vi "Transform.vi"(8 "error in (no error)":errorcluster caption="entrée d'erreur (pas d'erreur)", 9 "y":string[][](array[string]), 10 "X":string[][](array[string]), 11 "PowerTransformer.lvclass":refnum<class "PowerTransformer.lvclass">) -> (0 "error out":errorcluster caption="sortie d'erreur", 2 "Data":T1, 3 "PowerTransformer.lvclass":refnum<class "PowerTransformer.lvclass">)   [LabVIEW 2020, in "PowerTransformer.lvclass"]
doc: "Apply the power transform to each feature using the fitted lambdas.\n\nReturns : \n\n- X_trans : array-like, shape (n_samples, n_features)\nThe transformed data."
uses:
  PowerTransformer.lvclass
  PowerTransformer.lvclass/PowerTransformer.ctl
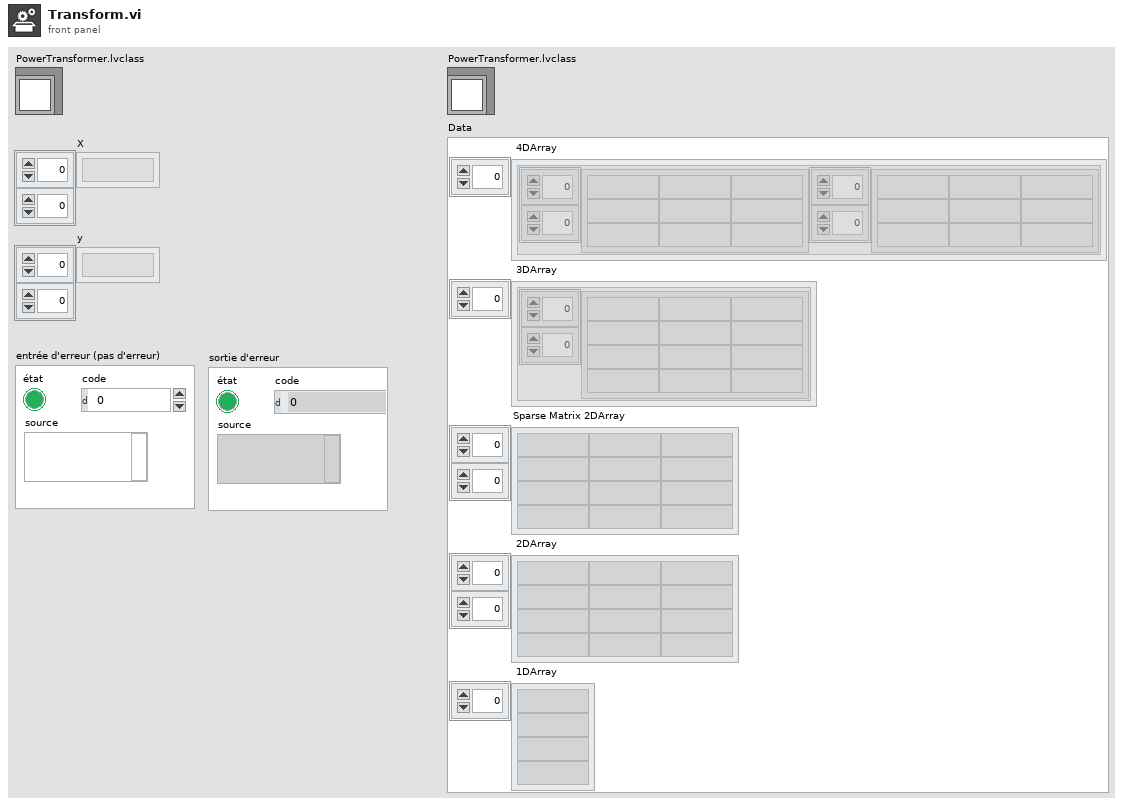
[diagram p1: front panel]
types:
  T1 = cluster{" 4DArray":cluster{"1":string[][], "2":string[][]}[], " 3DArray":cluster{"Tableau":string[][]}[], "Sparse Matrix 2DArray":string[][], " 2DArray":string[][], " 1DArray":string[]}
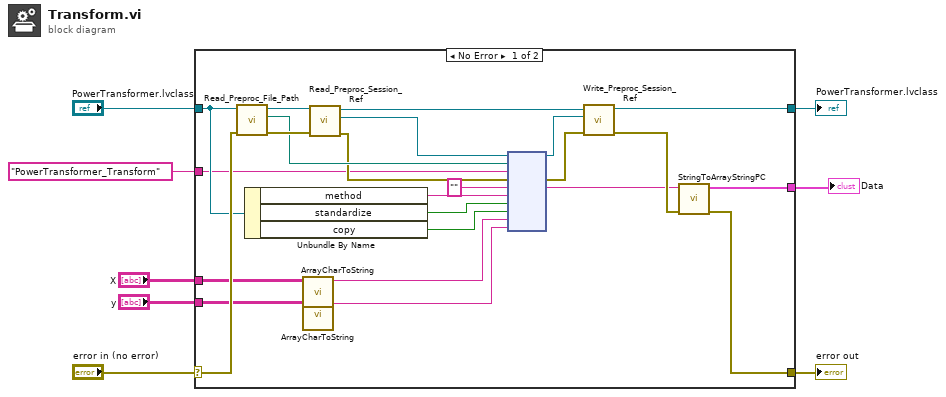
[diagram p0: block diagram]
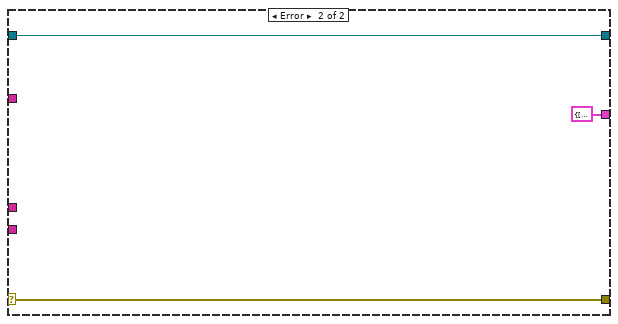
[diagram p2: hidden frame]
diagram:
  n1 = case shown="No Error" "error in (no error)" {
    selector: "error in (no error)" -> [w20 w35]
    tunnel: [w9 w35] -> w7
    tunnel: [w13 w34] -> w5
    tunnel: "PowerTransformer.lvclass" -> [w19 w34]
    tunnel: "PowerTransformer_Transform" ("Fonction") -> [w18 _]
    tunnel: [w10 T1 {" 4DArray"=[], " 3DArray"=[], "Sparse Matrix 2DArray"=[], " 2DArray"=[], " 1DArray"=[]} ("Data")] -> w3
    tunnel: "X" -> [w17 _]
    tunnel: "y" -> [w16 _]
    frame No Error {
      n2 = call-dynamic "Read_Preproc_File_Path.vi"("error in (no error)"=w20, "Python in"=w19) -> ("error out"=w31:errorcluster, "File_Path"=w28:path, "Python out"=w32:refnum<class "PowerTransformer.lvclass">)  [unwired: 7 in]
      n3 = Unbundle By Name(w19) -> ("method"=w23:string, "standardize"=w22:bool, "copy"=w21:bool)
      n4 = call "ArrayCharToString.vi"("TAB"=w17) -> ("Instruction"=w15:string)  [unwired: 10 in]
      n5 = call "ArrayCharToString.vi"("TAB"=w16) -> ("Instruction"=w14:string)  [unwired: 10 in]
      n6 = call-dynamic "Read_Preproc_Session_Ref.vi"("error in (no error)"=w31, "Python in"=w32) -> ("error out"=w27:errorcluster, "Session_ref"=w29:refnum<k35>, "Python out"=w30:refnum<class "PowerTransformer.lvclass">)  [unwired: 7 in]
      n7 = node(w29, w28, w18, w27, "", w23, w22, w21, w15, w14) -> (w25:refnum<k35>, w26:errorcluster, w11:string)  [unwired: 5 in, 2 out]
      n8 = call-dynamic "Write_Preproc_Session_Ref.vi"("error in (no error)"=w26, "Session_ref"=w25, "Python in"=w30) -> ("error out"=w12:errorcluster, "Python out"=w13:refnum<class "PowerTransformer.lvclass">)  [unwired: 7 in]
      n9 = call "StringToArrayStringPC.vi"("sortie d'erreur"=w12, "Return value"=w11) -> ("sortie d'erreur"=w9:errorcluster, "Data"=w10:T1)  [unwired: 8 in]
    }
    frame Error {
    }
  }
  "error out" <- w7
  "PowerTransformer.lvclass" <- w5
  "Data" <- w3
